vi "mqttCmdBuildFixedHeaderByte1.vi"(0 "retain(F)":bool, 1 "MessageType":T1, 5 "duplicate(F)":bool, 7 "QoS (At most once)":T2, 11 "error in (no error)":errorcluster) -> (4 "byte1":u8 format="%08b", 15 "error out":errorcluster)   [LabVIEW 2013, in "mqttCmd.lvclass"]
uses:
  mqttCmd.lvclass
  mqttTypedef/mqttQOSlevel.ctl
  mqttTypedef/mqttMessageType.ctl
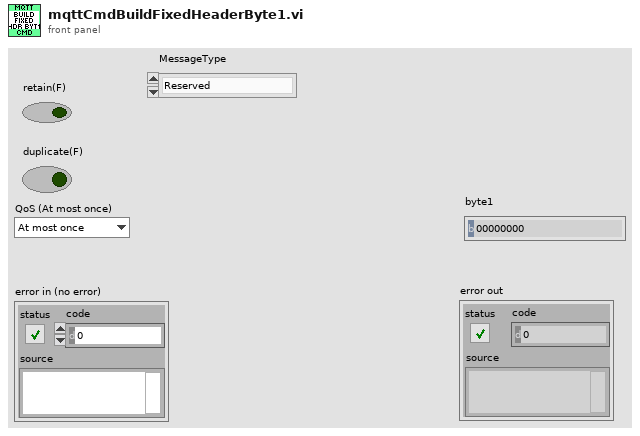
[diagram p1: front panel]
types:
  T1 = typedef "mqttMessageType.ctl" = enum32{"Reserved", "CONNECT", "CONNACK", "PUBLISH", "PUBACK", "PUBREC", "PUBREL", "PUBCOMP", "SUBSCRIBE", "SUBACK", "UNSUBSCRIBE", "UNSUBACK", "PINGREQ", "PINGRESP", "DISCONNECT", "Reserved2"}
  T2 = typedef "mqttQOSlevel.ctl" = enum8{"At most once", "At least once", "Exactly once", "Reserved"}
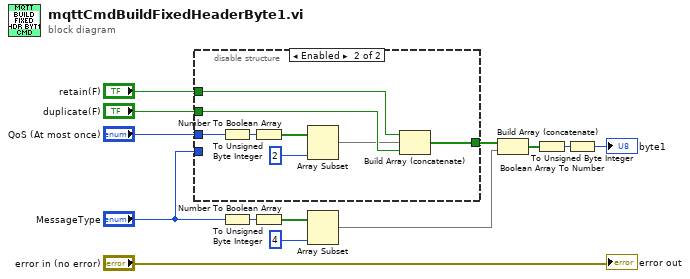
[diagram p0: block diagram]
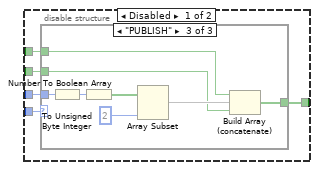
[diagram p2: hidden frame]
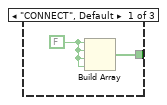
[diagram p3: hidden frame]
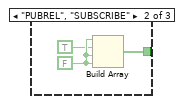
[diagram p4: hidden frame]
diagram:
  n1 = disable-structure shown="Enabled" {
    disable-tunnel: "duplicate(F)" -> [w18 w39]
    disable-tunnel: "QoS (At most once)" -> [w17 w38]
    disable-tunnel: "retain(F)" -> [w16 w37]
    disable-tunnel: [w15 w36] -> w9
    disable-tunnel: "MessageType" -> [w14 _]
    frame Disabled {
      n2 = case shown="\"PUBLISH\"" w14 {
        tunnel: [w20 w23 w31] -> w15
        tunnel: w16 -> [_ _ w30]
        tunnel: w17 -> [_ _ w28]
        tunnel: w18 -> [_ _ w24]
        frame "CONNECT", Default {
          w19 = FALSE
          n3 = Build Array(w19, w19, w19, w19) -> (w20:bool[])
        }
        frame "PUBREL", "SUBSCRIBE" {
          w22 = FALSE
          n4 = Build Array(w22, TRUE, w22, w22) -> (w23:bool[])
        }
        frame "PUBLISH" {
          n5 = To Unsigned Byte Integer(number=w28) -> (unsigned 8bit integer=w29:u8)
          n6 = Number To Boolean Array(number=w29) -> (Boolean array=w27:bool[])
          n7 = Array Subset(array=w27, length=2) -> (w25:bool[])  [unwired: 1 in]
          n8 = Build Array (concatenate)(w30, w25, w24) -> (w31:bool[])
        }
      }
    }
    frame Enabled {
      n9 = To Unsigned Byte Integer(number=w38) -> (unsigned 8bit integer=w35:u8)
      n10 = Number To Boolean Array(number=w35) -> (Boolean array=w34:bool[])
      n11 = Array Subset(array=w34, length=2) -> (w32:bool[])  [unwired: 1 in]
      n12 = Build Array (concatenate)(w37, w32, w39) -> (w36:bool[])
    }
  }
  n13 = To Unsigned Byte Integer(number="MessageType") -> (unsigned 8bit integer=w7:u8)
  n14 = Number To Boolean Array(number=w7) -> (Boolean array=w5:bool[])
  n15 = Array Subset(array=w5, length=4) -> (w2:bool[])  [unwired: 1 in]
  n16 = Build Array (concatenate)(w9, w2) -> (w10:bool[])
  n17 = Boolean Array To Number(Boolean array=w10) -> (number=w8:u32)
  n18 = To Unsigned Byte Integer(number=w8) -> (unsigned 8bit integer=→"byte1":u8)
  "error out" <- "error in (no error)"
